vi "wait.vi"(1 "error in (no error)":errorcluster, 2 "wait time (ms)":i32=1) -> (0 "error in (no error) 2":errorcluster)   [LabVIEW 2011]
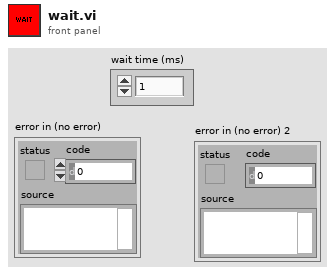
[diagram p1: front panel]
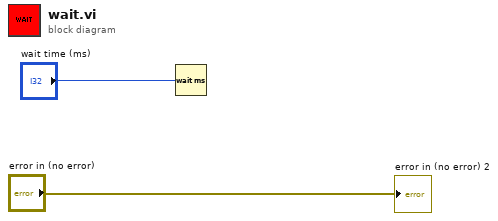
[diagram p0: block diagram]
diagram:
  n1 = Wait (ms)(milliseconds to wait="wait time (ms)") -> ()  [unwired: 1 out]
  "error in (no error) 2" <- "error in (no error)"
